vi "Display_HGB2.vi"(0 "data":waveform(dbl)[](array[waveform])=[{"t0"=timestamp(3711548043.869262 s since 1904-01-01), "dt"=0.1, "Y"=[28.025140044852478, 28.025140044852478, 28.025140044852478, 28.025140044852478, 28.025140044852478], "attributes"=variant("NI_ChannelName"=variant(string "T_dis_dwnstrm"), "NI_UnitDescription"=variant(string "Deg C"))}, {"t0"=timestamp(3711548043.869262 s since 1904-01-01), "dt"=0.1, "Y"=[27.82403761388044, 27.82403761388044, 27.82403761388044, 27.82403761388044, 27.82403761388044], "attributes"=variant("NI_ChannelName"=variant(string "T_liq_mix"), "NI_UnitDescription"=variant(string "Deg C"))}, {"t0"=timestamp(3711548043.869262 s since 1904-01-01), "dt"=0.1, "Y"=[27.478899133975307, 27.478899133975307, 27.478899133975307, 27.478899133975307, 27.478899133975307], "attributes"=variant("NI_ChannelName"=variant(string "T_gas_mix"), "NI_UnitDescription"=variant(string "Deg C"))}, {"t0"=timestamp(3711548043.869262 s since 1904-01-01), "dt"=0.1, "Y"=[27.84040164299891, 27.84040164299891, 27.84040164299891, 27.84040164299891, 27.84040164299891], "attributes"=variant("NI_ChannelName"=variant(string "T_wf_cond_out"), "NI_UnitDescription"=variant(string "Deg C"))}, {"t0"=timestamp(3711548043.869262 s since 1904-01-01), "dt"=0.1, "Y"=[27.706063700548942, 27.706063700548942, 27.706063700548942, 27.706063700548942, 27.706063700548942], "attributes"=variant("NI_ChannelName"=variant(string "T_cf_in"), "NI_UnitDescription"=variant(string "Deg C"))}, {"t0"=timestamp(3711548043.869262 s since 1904-01-01), "dt"=0.1, "Y"=[27.72811498240912, 27.72811498240912, 27.72811498240912, 27.72811498240912, 27.72811498240912], "attributes"=variant("NI_ChannelName"=variant(string "T_comp_suc"), "NI_UnitDescription"=variant(string "Deg C"))}, {"t0"=timestamp(3711548043.869262 s since 1904-01-01), "dt"=0.1, "Y"=[27.186769428501513, 27.186769428501513, 27.186769428501513, 27.186769428501513, 27.186769428501513], "attributes"=variant("NI_ChannelName"=variant(string "T_comp_dis"), "NI_UnitDescription"=variant(string "Deg C"))}, {"t0"=timestamp(3711548043.869262 s since 1904-01-01), "dt"=0.1, "Y"=[-58035.88440566614, -58035.88440566614, -58035.88440566614, -58035.88440566614, -58035.88440566614], "attributes"=variant("NI_ChannelName"=variant(string "NC3"), "NI_UnitDescription"=variant(string "Deg C"))}, {"t0"=timestamp(3711548043.869262 s since 1904-01-01), "dt"=0.1, "Y"=[-58035.88440566614, -58035.88440566614, -58035.88440566614, -58035.88440566614, -58035.88440566614], "attributes"=variant("NI_ChannelName"=variant(string "NC4"), "NI_UnitDescription"=variant(string "Deg C"))}, {"t0"=timestamp(3711548043.869262 s since 1904-01-01), "dt"=0.1, "Y"=[-58035.88440566614, -58035.88440566614, -58035.88440566614, -58035.88440566614, -58035.88440566614], "attributes"=variant("NI_ChannelName"=variant(string "NC5"), "NI_UnitDescription"=variant(string "Deg C"))}, {"t0"=timestamp(3711548043.869262 s since 1904-01-01), "dt"=0.1, "Y"=[-58035.88440566614, -58035.88440566614, -58035.88440566614, -58035.88440566614, -58035.88440566614], "attributes"=variant("NI_ChannelName"=variant(string "NC6"), "NI_UnitDescription"=variant(string "Deg C"))}, {"t0"=timestamp(3711548043.869262 s since 1904-01-01), "dt"=0.1, "Y"=[-58035.88440566614, -58035.88440566614, -58035.88440566614, -58035.88440566614, -58035.88440566614], "attributes"=variant("NI_ChannelName"=variant(string "NC7"), "NI_UnitDescription"=variant(string "Deg C"))}, {"t0"=timestamp(3711548043.869262 s since 1904-01-01), "dt"=0.1, "Y"=[-58035.88440566614, -58035.88440566614, -58035.88440566614, -58035.88440566614, -58035.88440566614], "attributes"=variant("NI_ChannelName"=variant(string "NC8"), "NI_UnitDescription"=variant(string "Deg C"))}, {"t0"=timestamp(3711548043.869262 s since 1904-01-01), "dt"=0.1, "Y"=[-58035.88440566614, -58035.88440566614, -58035.88440566614, -58035.88440566614, -58035.88440566614], "attributes"=variant("NI_ChannelName"=variant(string "NC9"), "NI_UnitDescription"=variant(string "Deg C"))}, {"t0"=timestamp(3711548043.869262 s since 1904-01-01), "dt"=0.1, "Y"=[-58035.88440566614, -58035.88440566614, -58035.88440566614, -58035.88440566614, -58035.88440566614], "attributes"=variant("NI_ChannelName"=variant(string "NC10"), "NI_UnitDescription"=variant(string "Deg C"))}, {"t0"=timestamp(3711548043.869262 s since 1904-01-01), "dt"=0.1, "Y"=[-58035.88440566614, -58035.88440566614, -58035.88440566614, -58035.88440566614, -58035.88440566614], "attributes"=variant("NI_ChannelName"=variant(string "NC11"), "NI_UnitDescription"=variant(string "Deg C"))}, {"t0"=timestamp(3711548043.869262 s since 1904-01-01), "dt"=0.1, "Y"=[714.515263053155, 714.5034308747695, 714.4757097711235, 714.5010644390925, 714.5199959245092], "attributes"=variant("NI_ChannelName"=variant(string "P_comp_suc"))}, {"t0"=timestamp(3711548043.869262 s since 1904-01-01), "dt"=0.1, "Y"=[714.711979590679, 714.6382820224494, 714.6328730266159, 714.6423387693244, 714.687639109429], "attributes"=variant("NI_ChannelName"=variant(string "P_comp_dis"))}, {"t0"=timestamp(3711548043.869262 s since 1904-01-01), "dt"=0.1, "Y"=[714.5751000695618, 714.7066062807608, 714.6815896750313, 714.6481215133124, 714.5676627002908], "attributes"=variant("NI_ChannelName"=variant(string "P_comp_int"))}, {"t0"=timestamp(3711548043.869262 s since 1904-01-01), "dt"=0.1, "Y"=[-2.0166503493911775e-05, -2.024005106758542e-05, -2.028908278336669e-05, -2.0252308996531604e-05, -2.0252308996531604e-05], "attributes"=variant("NI_ChannelName"=variant(string "m_dot_wf"))}, {"t0"=timestamp(3711548043.869262 s since 1904-01-01), "dt"=0.1, "Y"=[-0.03114398103542726, -0.03114398103542726, -0.030996885888072256, -0.03094785417229673, -0.03134010789855779], "attributes"=variant("NI_ChannelName"=variant(string "Voltage"))}, {"t0"=timestamp(3711548043.869262 s since 1904-01-01), "dt"=0.1, "Y"=[-0.026643512746304054, -0.026708888367345196, -0.026692544462086687, -0.026447385883173524, -0.026692544462086687], "attributes"=variant("NI_ChannelName"=variant(string "Frequency"))}, {"t0"=timestamp(3711548043.869262 s since 1904-01-01), "dt"=0.1, "Y"=[1.2552119240291074e-06, 1.2159865514031977e-06, 1.2159865514031977e-06, 1.150610930360015e-06, 1.124460681942742e-06], "attributes"=variant("NI_ChannelName"=variant(string "NC12"))}, {"t0"=timestamp(3711548043.869262 s since 1904-01-01), "dt"=0.1, "Y"=[-0.0010623538419517185, -0.0010623538419517185, -0.0011277294629949012, -0.0011440733682556968, -0.0011604172735164926], "attributes"=variant("NI_ChannelName"=variant(string "NC13"))}], 7 "NI 6001":waveform(dbl)[](array[waveform])=[{"t0"=timestamp(3711548043.5702925 s since 1904-01-01), "dt"=0.1, "Y"=[0.02366427518427372, 0.03397996537387371, 0.03397996537387371, 0.039137810468673706, 0.039137810468673706], "attributes"=variant("NI_ChannelName"=variant(string "Torque"))}, {"t0"=timestamp(3711548043.620291 s since 1904-01-01), "dt"=0.1, "Y"=[-7.039394229650497, 5.339433997869492, -11.165670305490494, 1.2131579220294952, -0.8499801158905029], "attributes"=variant("NI_ChannelName"=variant(string "Tachometer"))}], 11 "error in (no error)":errorcluster) -> (2 "Mass Flow":waveform(dbl)={"t0"=timestamp(3711548043.869262 s since 1904-01-01), "dt"=0.1, "Y"=[-2.0166503493911775e-05, -2.024005106758542e-05, -2.028908278336669e-05, -2.0252308996531604e-05, -2.0252308996531604e-05], "attributes"=variant("NI_ChannelName"=variant(string "m_dot_wf"))}, 4 "System Pressures":waveform(dbl)[](array[waveform])=[{"t0"=timestamp(3711548043.869262 s since 1904-01-01), "dt"=0.1, "Y"=[714.515263053155, 714.5034308747695, 714.4757097711235, 714.5010644390925, 714.5199959245092], "attributes"=variant("NI_ChannelName"=variant(string "P_comp_suc"))}, {"t0"=timestamp(3711548043.869262 s since 1904-01-01), "dt"=0.1, "Y"=[714.711979590679, 714.6382820224494, 714.6328730266159, 714.6423387693244, 714.687639109429], "attributes"=variant("NI_ChannelName"=variant(string "P_comp_dis"))}, {"t0"=timestamp(3711548043.869262 s since 1904-01-01), "dt"=0.1, "Y"=[714.5751000695618, 714.7066062807608, 714.6815896750313, 714.6481215133124, 714.5676627002908], "attributes"=variant("NI_ChannelName"=variant(string "P_comp_int"))}], 6 "Data Array":dbl[](array[numeric])=[28.02514004485248, 27.82403761388044, 27.478899133975307, 27.84040164299891, 27.706063700548942, 27.728114982409117, 27.186769428501513, -58035.88440566613, -58035.88440566613, -58035.88440566613, -58035.88440566613, -58035.88440566613, -58035.88440566613, -58035.88440566613, -58035.88440566613, -58035.88440566613, 714.50309281253, 714.6626225036995, 714.6358160477914, -2.024005106758542e-05, -0.031114562005956258, -0.02663697518419923, 1.1924513278276517e-06, -0.0011113855577341055, 0.02366427518427372, 0.03397996537387371, 0.03397996537387371, 0.039137810468673706, 0.039137810468673706, -7.039394229650497, 5.339433997869492, -11.165670305490494, 1.2131579220294952, -0.8499801158905029], 8 "Power Constituents":waveform(dbl)[](array[waveform])=[{"t0"=timestamp(3711548043.869262 s since 1904-01-01), "dt"=0.1, "Y"=[-0.03114398103542726, -0.03114398103542726, -0.030996885888072256, -0.03094785417229673, -0.03134010789855779], "attributes"=variant("NI_ChannelName"=variant(string "Voltage"))}, {"t0"=timestamp(3711548043.869262 s since 1904-01-01), "dt"=0.1, "Y"=[-0.026643512746304054, -0.026708888367345196, -0.026692544462086687, -0.026447385883173524, -0.026692544462086687], "attributes"=variant("NI_ChannelName"=variant(string "Frequency"))}, {"t0"=timestamp(3711548043.5702925 s since 1904-01-01), "dt"=0.1, "Y"=[0.02366427518427372, 0.03397996537387371, 0.03397996537387371, 0.039137810468673706, 0.039137810468673706], "attributes"=variant("NI_ChannelName"=variant(string "Torque"))}, {"t0"=timestamp(3711548043.620291 s since 1904-01-01), "dt"=0.1, "Y"=[-7.039394229650497, 5.339433997869492, -11.165670305490494, 1.2131579220294952, -0.8499801158905029], "attributes"=variant("NI_ChannelName"=variant(string "Tachometer"))}], 10 "Setpoint Temperatures":waveform(dbl)[](array[waveform])=[{"t0"=timestamp(3711548043.869262 s since 1904-01-01), "dt"=0.1, "Y"=[27.72811498240912, 27.72811498240912, 27.72811498240912, 27.72811498240912, 27.72811498240912], "attributes"=variant("NI_ChannelName"=variant(string "T_comp_suc"), "NI_UnitDescription"=variant(string "Deg C"))}, {"t0"=timestamp(3711548043.869262 s since 1904-01-01), "dt"=0.1, "Y"=[27.186769428501513, 27.186769428501513, 27.186769428501513, 27.186769428501513, 27.186769428501513], "attributes"=variant("NI_ChannelName"=variant(string "T_comp_dis"), "NI_UnitDescription"=variant(string "Deg C"))}, {"t0"=timestamp(0 s since 1904-01-01), "dt"=1.0, "Y"=[0.366537967906023, 0.3671027106300322, 0.36842584966040803, 0.367215660017731, 0.36631207278304245], "attributes"=variant("NI_ChannelName"=variant(string "Suc_Suph"))}], 12 "error out":errorcluster, 15 "System Temperatures":waveform(dbl)[](array[waveform])=[{"t0"=timestamp(3711548043.869262 s since 1904-01-01), "dt"=0.1, "Y"=[28.025140044852478, 28.025140044852478, 28.025140044852478, 28.025140044852478, 28.025140044852478], "attributes"=variant("NI_ChannelName"=variant(string "T_dis_dwnstrm"), "NI_UnitDescription"=variant(string "Deg C"))}, {"t0"=timestamp(3711548043.869262 s since 1904-01-01), "dt"=0.1, "Y"=[27.82403761388044, 27.82403761388044, 27.82403761388044, 27.82403761388044, 27.82403761388044], "attributes"=variant("NI_ChannelName"=variant(string "T_liq_mix"), "NI_UnitDescription"=variant(string "Deg C"))}, {"t0"=timestamp(3711548043.869262 s since 1904-01-01), "dt"=0.1, "Y"=[27.478899133975307, 27.478899133975307, 27.478899133975307, 27.478899133975307, 27.478899133975307], "attributes"=variant("NI_ChannelName"=variant(string "T_gas_mix"), "NI_UnitDescription"=variant(string "Deg C"))}, {"t0"=timestamp(3711548043.869262 s since 1904-01-01), "dt"=0.1, "Y"=[27.84040164299891, 27.84040164299891, 27.84040164299891, 27.84040164299891, 27.84040164299891], "attributes"=variant("NI_ChannelName"=variant(string "T_wf_cond_out"), "NI_UnitDescription"=variant(string "Deg C"))}, {"t0"=timestamp(3711548043.869262 s since 1904-01-01), "dt"=0.1, "Y"=[27.706063700548942, 27.706063700548942, 27.706063700548942, 27.706063700548942, 27.706063700548942], "attributes"=variant("NI_ChannelName"=variant(string "T_cf_in"), "NI_UnitDescription"=variant(string "Deg C"))}])   [LabVIEW 2016]
uses:
  <vilib>/Utility/error.llb/DialogType.ctl
panel:
  out "Double Array Empty?":bool
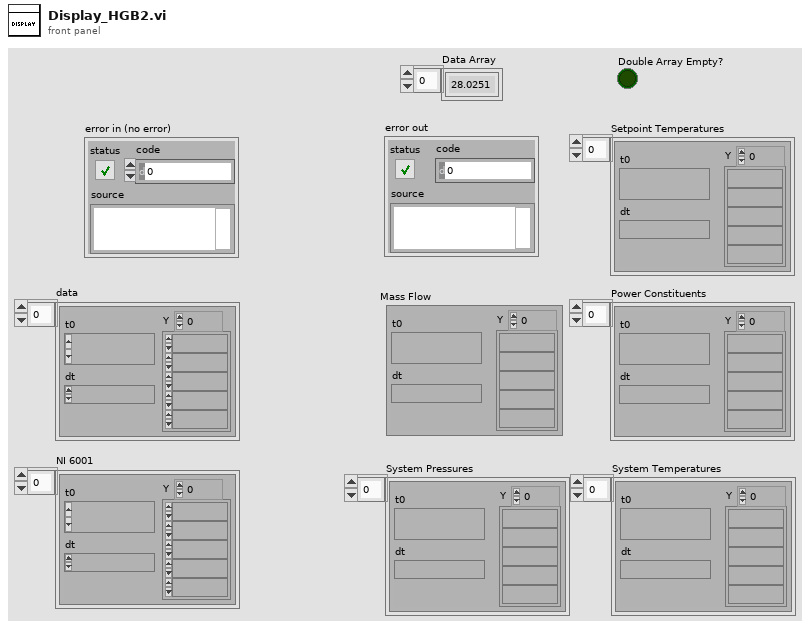
[diagram p1: front panel]
types:
  T1 = typedef "DialogType.ctl" = u16
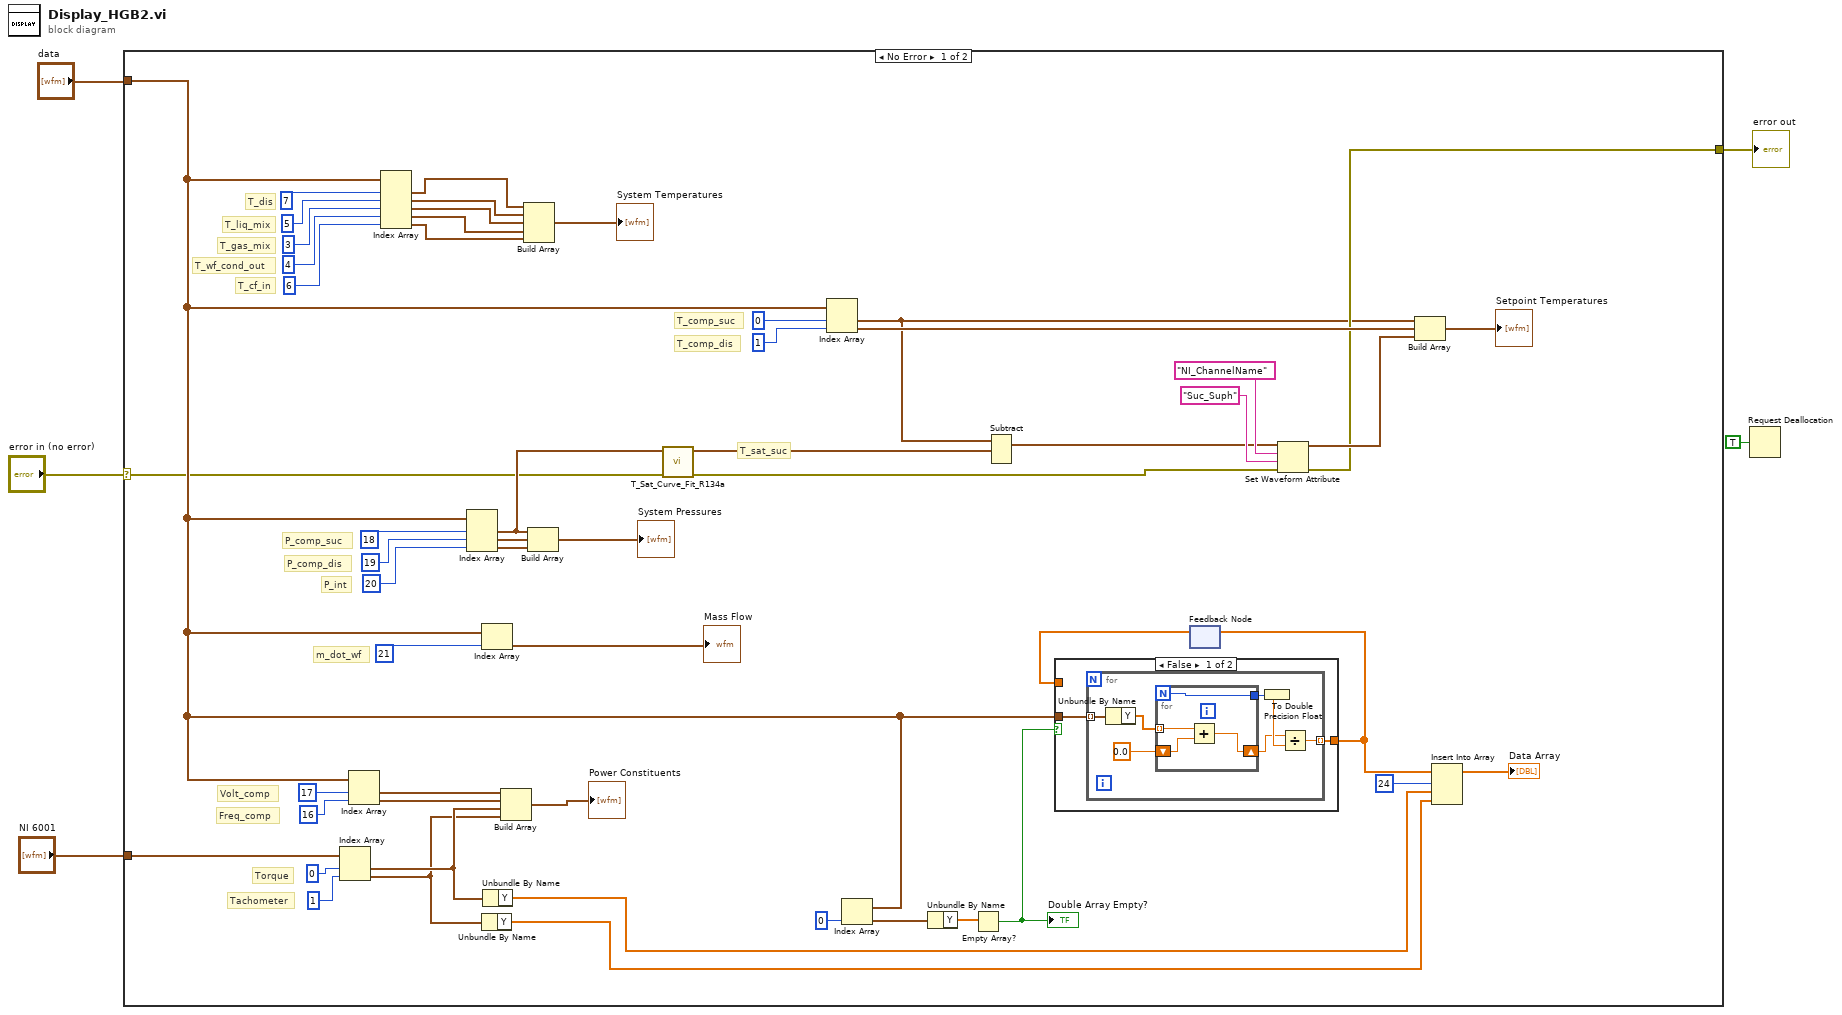
[diagram p0: block diagram]
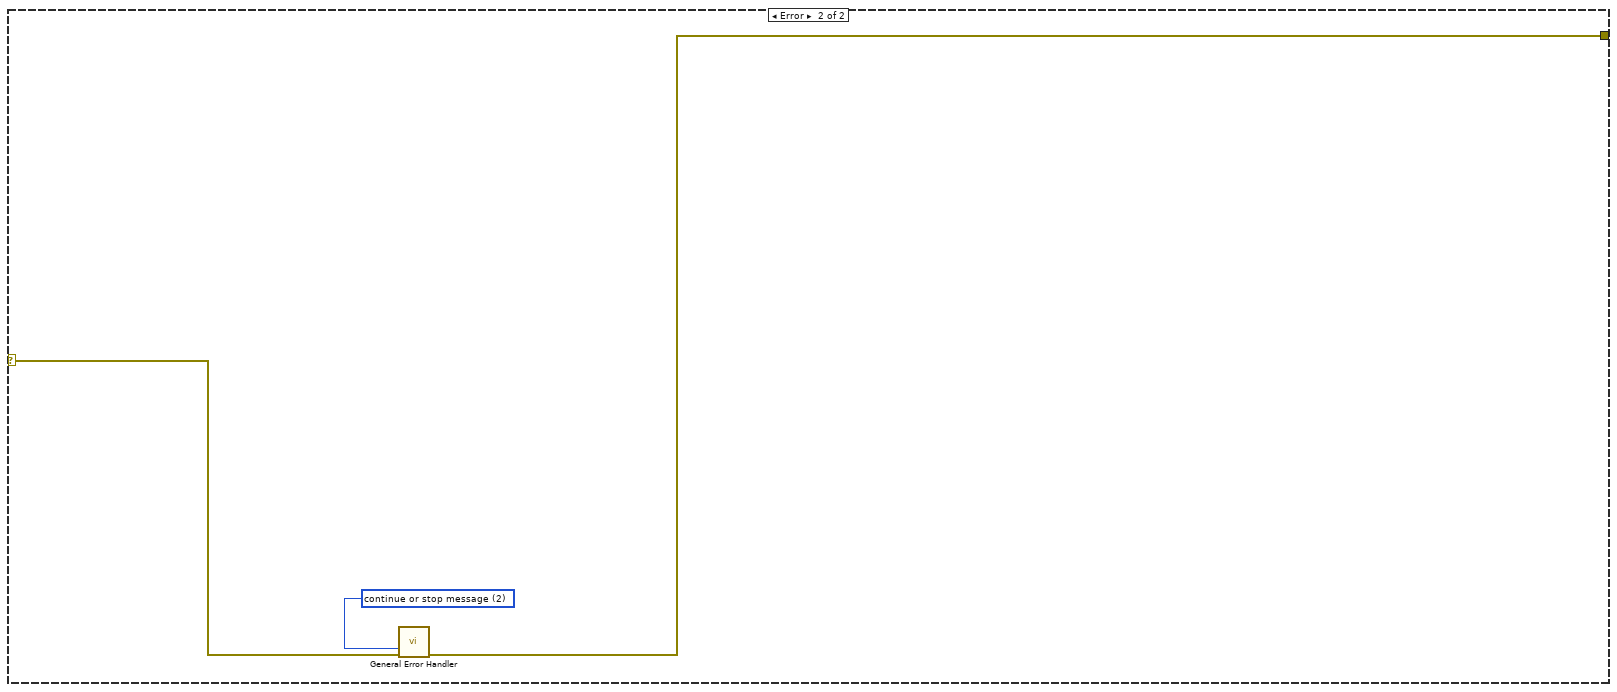
[diagram p3: hidden frame]
diagram:
  n1 = case shown="No Error" "error in (no error)" {
    selector: "error in (no error)" -> [w6 w74]
    tunnel: "data" -> [w19 _]
    tunnel: [w12 w75] -> w3
    tunnel: "NI 6001" -> [w35 _]
    frame No Error {
      # "T_sat_suc"
      # "T_comp_dis"
      # "T_comp_suc"
      # "Tachometer"
      # "Torque"
      # "m_dot_wf"
      # "P_int"
      # "P_comp_dis"
      # "P_comp_suc"
      # "Freq_comp"
      # "Volt_comp"
      # "T_cf_in"
      # "T_wf_cond_out"
      # "T_gas_mix"
      # "T_liq_mix"
      # "T_dis"
      n2 = Index Array(array=w35, index #1=0 ("index"), index #2=1 ("index")) -> (element #1=w27:waveform(dbl), element #2=w22:waveform(dbl))
      n3 = Index Array(array=w19, index #1=17 ("index"), index #2=16 ("index")) -> (element #1=w50:waveform(dbl), element #2=w51:waveform(dbl))
      n4 = Index Array(array=w19, index #1=7 ("index"), index #2=5 ("index"), index #3=3 ("index"), index #4=4 ("index"), index #5=6 ("index")) -> (element #1=w49:waveform(dbl), element #2=w44:waveform(dbl), element #3=w48:waveform(dbl), element #4=w47:waveform(dbl), element #5=w46:waveform(dbl))
      n5 = Index Array(array=w19, index #1=18 ("index"), index #2=19 ("index"), index #3=20 ("index")) -> (element #1=w10:waveform(dbl), element #2=w39:waveform(dbl), element #3=w40:waveform(dbl))
      n6 = Index Array(array=w19, index=21) -> (element=→"Mass Flow":waveform(dbl))
      n7 = Unbundle By Name(w22) -> ("Y"=w24:dbl[])
      n8 = Unbundle By Name(w27) -> ("Y"=w26:dbl[])
      n9 = Build Array(w50, w51, w27, w22) -> (→"Power Constituents":waveform(dbl)[])
      n10 = Build Array(w49, w44, w48, w47, w46) -> (→"System Temperatures":waveform(dbl)[])
      n11 = Build Array(w10, w39, w40) -> (→"System Pressures":waveform(dbl)[])
      n12 = call "T_Sat_Curve_Fit_R134a.vi"("error in (no error)"=w6, "Waveform in"=w10) -> ("error out"=w7:errorcluster, "Waveform out"=w9:waveform(dbl))  [unwired: 8 in]
      n13 = Index Array(array=w19, index #1=0 ("index"), index #2=1 ("index")) -> (element #1=w11:waveform(dbl), element #2=w20:waveform(dbl))
      n14 = Index Array(array=w19, index=0) -> (element=w32:waveform(dbl))
      n15 = Unbundle By Name(w32) -> ("Y"=w31:dbl[])
      n16 = Empty Array?(array=w31) -> (empty?=w30:bool)
      "Double Array Empty?" <- w30
      n17 = Subtract(1:w9, 2:w11) -> (0:w8:waveform(dbl))  [unwired: 1 in, 1 out]
      n18 = feedback #1() -> (w34:dbl[])  [unwired: 1 in]
      n19 = case shown="False" w30 {
        tunnel: w19 -> [w61 _]
        tunnel: [w60 w73] -> w29
        tunnel: w34 -> [_ w73]
        frame False {
          n20 = for {
            tunnel: w61 -> [w68] mode=indexing
            tunnel: [w62] -> w60 mode=indexing
            n21 = Unbundle By Name(w68) -> ("Y"=w66:dbl[])
            n22 = for {
              N -> [w70]
              shift-right: [w69] -> w63
              shift-left: 0.0 -> [w72]
              tunnel: w66 -> [w71] mode=indexing
              tunnel: [w70] -> w65
              n23 = Add(x=w71, y=w72) -> (x+y=w69:dbl)
            }
            n24 = To Double Precision Float(number=w65) -> (double precision float=w64:dbl)
            n25 = Divide(x=w63, y=w64) -> (x/y=w62:dbl)
          }
        }
        frame True {
        }
      }
      n26 = feedback-in #1(w29) -> ()
      n27 = Set Waveform Attribute(4:w7, 5:"Suc_Suph" ("name"), 6:"NI_ChannelName" ("name"), 7:w8) -> (0:w12:errorcluster, 3:w13:waveform(dbl))  [unwired: 1 out]
      n28 = Build Array(w11, w20, w13) -> (→"Setpoint Temperatures":waveform(dbl)[])
      n29 = Insert Into Array(array=w29, index=24, new element #1=w26, new element #2=w24) -> (→"Data Array":dbl[])
    }
    frame Error {
      w76 = T1 2 items=["no dialog", "OK message", "continue or stop message", "OK message + warnings", "continue/stop + warnings"] ("type of dialog (OK msg:1)")
      n30 = call <vilib>:"General Error Handler.vi"("type of dialog (OK msg:1)"=w76, "error in (no error)"=w74) -> ("error out"=w75:errorcluster)  [unwired: 9 in, 4 out]
    }
  }
  "error out" <- w3
  n31 = Request Deallocation(TRUE ("flag")) -> ()
